vi "FilterBySizeAndColor.vi"(9 "Color":T1, 10 "Size":T2, 11 "Products In":refnum<class "Product.lvclass">[](array[class])) -> (3 "Filtered Products":refnum<class "Product.lvclass">[](array[class]))   [LabVIEW 2018, in "ProductFilter.lvclass"]
uses:
  ProductFilter.lvclass
  Product/Product.lvclass
  Product/Size.ctl
  Product/Color.ctl
  Product/Product.lvclass/Product.ctl
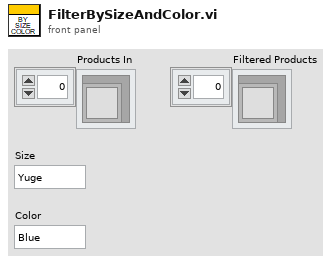
[diagram p1: front panel]
types:
  T1 = typedef "Product.lvclass/Color.ctl" = enum16{"Blue", "Green", "Red"}
  T2 = typedef "Product.lvclass/Size.ctl" = enum16{"Yuge", "Big", "Medium", "Small"}
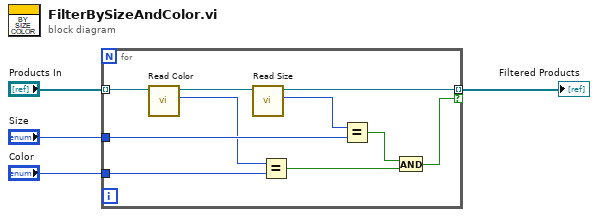
[diagram p0: block diagram]
diagram:
  n1 = for {
    tunnel: "Products In" -> [w11] mode=indexing
    tunnel: [w13] -> w3 mode=indexing if=w5
    tunnel: "Size" -> [w14]
    tunnel: "Color" -> [w8]
    n2 = call "Read Color.vi"("Product In"=w11) -> ("Color"=w9:T1, "Product Out"=w10:refnum<class "Product.lvclass">)  [unwired: 9 in]
    n3 = call "Read Size.vi"("Product In"=w10) -> ("Size"=w12:T2, "Product Out"=w13:refnum<class "Product.lvclass">)  [unwired: 9 in]
    n4 = Equal?(x=w9, y=w8) -> (x = y?=w7:bool)
    n5 = Equal?(x=w12, y=w14) -> (x = y?=w6:bool)
    n6 = And(x=w6, y=w7) -> (x .and. y?=w5:bool)
  }
  "Filtered Products" <- w3
